vi "1SDI_MaxMin_v00.vi"(8 "Reset MaxMin?":T2, 9 "Min (-1)":T3, 10 "Max (-1)":T4, 11 "Graph Errors":T1) -> (0 "Max":T4, 3 "Min":T3)   [LabVIEW 2011]
uses:
  Strict Type Defs/1SDI Max.ctl
  Strict Type Defs/1SDI Min.ctl
  Strict Type Defs/1SDI Reset MaxMin.ctl
  Strict Type Defs/Error Signals 1SDI.ctl
panel:
  in  "Min typedef":T3
  in  "Max typedef":T4
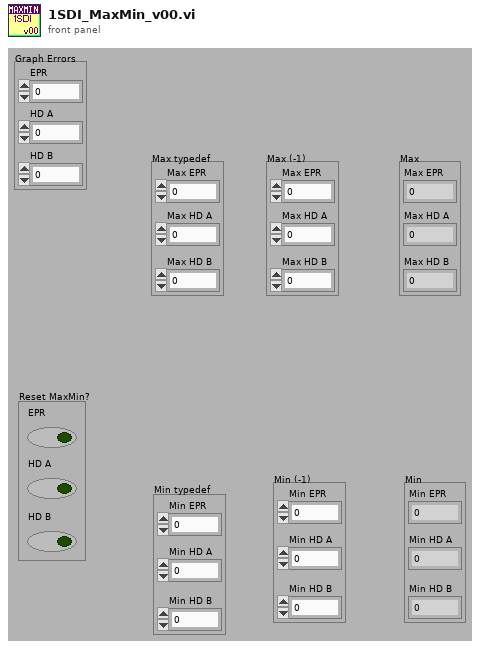
[diagram p1: front panel]
types:
  T1 = typedef "Error Signals 1SDI.ctl" = cluster{"EPR":i16, "HD A":i16, "HD B":i16}
  T2 = typedef "1SDI Reset MaxMin.ctl" = cluster{"EPR":bool, "HD A":bool, "HD B":bool}
  T3 = typedef "1SDI Min.ctl" = cluster{"Min EPR":i16, "Min HD A":i16, "Min HD B":i16}
  T4 = typedef "1SDI Max.ctl" = cluster{"Max EPR":i16, "Max HD A":i16, "Max HD B":i16}
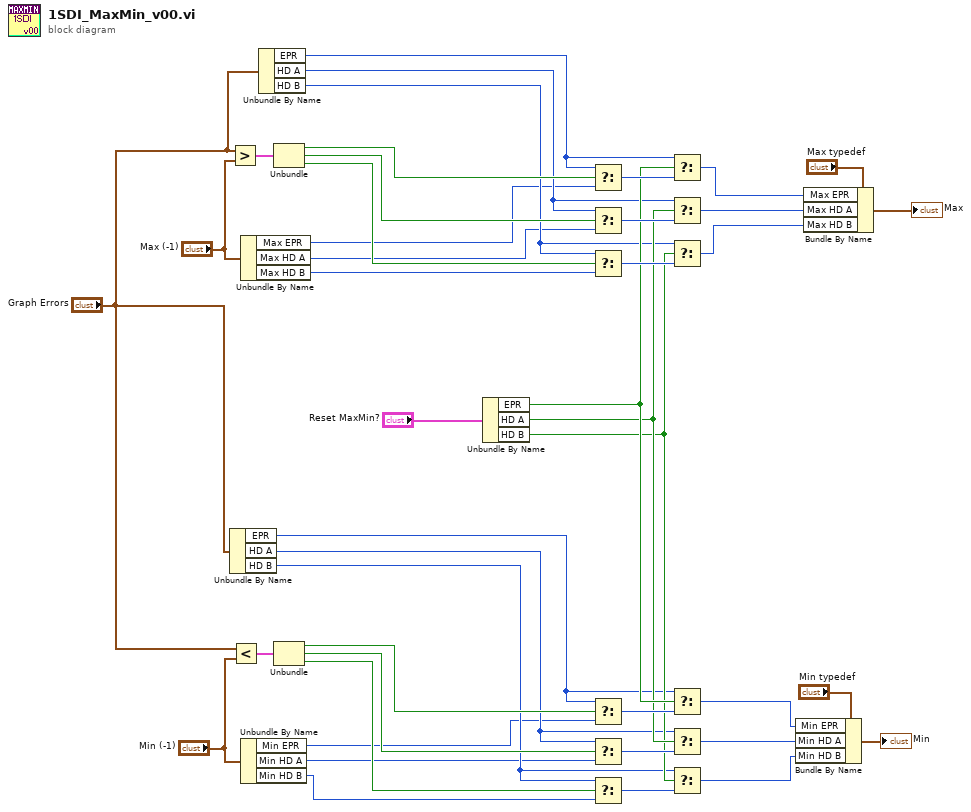
[diagram p0: block diagram]
diagram:
  n1 = Greater?(x="Graph Errors", y="Max (-1)") -> (0:w42:cluster{bool, bool, bool})
  n2 = Unbundle By Name("Graph Errors") -> ("EPR"=w11:i16, "HD A"=w10:i16, "HD B"=w9:i16)
  n3 = Less?(x="Graph Errors", y="Min (-1)") -> (x < y?=w38:cluster{bool, bool, bool})
  n4 = Unbundle By Name("Max (-1)") -> ("Max EPR"=w16:i16, "Max HD A"=w17:i16, "Max HD B"=w18:i16)
  n5 = Unbundle By Name("Min (-1)") -> ("Min EPR"=w8:i16, "Min HD A"=w7:i16, "Min HD B"=w6:i16)
  n6 = Unbundle By Name("Graph Errors") -> ("EPR"=w20:i16, "HD A"=w21:i16, "HD B"=w22:i16)
  n7 = Unbundle(w42) -> (w32:bool, w31:bool, w30:bool)
  n8 = Unbundle(w38) -> (w14:bool, w13:bool, w12:bool)
  n9 = Unbundle By Name("Reset MaxMin?") -> ("EPR"=w29:bool, "HD A"=w28:bool, "HD B"=w27:bool)
  n10 = Select(t=w20, s=w32, f=w16) -> (s? t:f=w41:i16)
  n11 = Select(t=w21, s=w31, f=w17) -> (s? t:f=w33:i16)
  n12 = Select(t=w22, s=w30, f=w18) -> (s? t:f=w34:i16)
  n13 = Select(t=w11, s=w14, f=w8) -> (s? t:f=w39:i16)
  n14 = Select(t=w10, s=w13, f=w7) -> (s? t:f=w36:i16)
  n15 = Select(t=w9, s=w12, f=w6) -> (s? t:f=w35:i16)
  n16 = Select(t=w20, s=w29, f=w41) -> (s? t:f=w25:i16)
  n17 = Select(t=w21, s=w28, f=w33) -> (s? t:f=w26:i16)
  n18 = Select(t=w22, s=w27, f=w34) -> (s? t:f=w24:i16)
  n19 = Select(t=w11, s=w29, f=w39) -> (s? t:f=w3:i16)
  n20 = Select(t=w10, s=w28, f=w36) -> (s? t:f=w2:i16)
  n21 = Select(t=w9, s=w27, f=w35) -> (s? t:f=w1:i16)
  n22 = Bundle By Name(cluster="Min typedef", "Min EPR"=w3, "Min HD A"=w2, "Min HD B"=w1) -> (→"Min":T3)
  n23 = Bundle By Name(cluster="Max typedef", "Max EPR"=w25, "Max HD A"=w26, "Max HD B"=w24) -> (→"Max":T4)
